vi "Quadro.vi"() -> ()   [LabVIEW 2012]
panel:
  out "Kąt x 2":u32
  out "Kąt x":u32
  out "Kąt y 2":u32
  out "Kąt y":u32
  out "Kąt z 2":u32
  out "Kąt z":u32
  out "x+y":u16
  out "Array":u8[](array[numeric])
  in  "Stop":bool
  out "error out":errorcluster
  in  "Opóźnienie pętli [ms]":u32
  in  "Czas oczekiwania po wysłaniu [ms]":u32
  in  "Dane wysłane":string="d"
  out "Nazwa urządzenia":string
  in  "Limit czasu - bluetooth [ms]":i32=1000
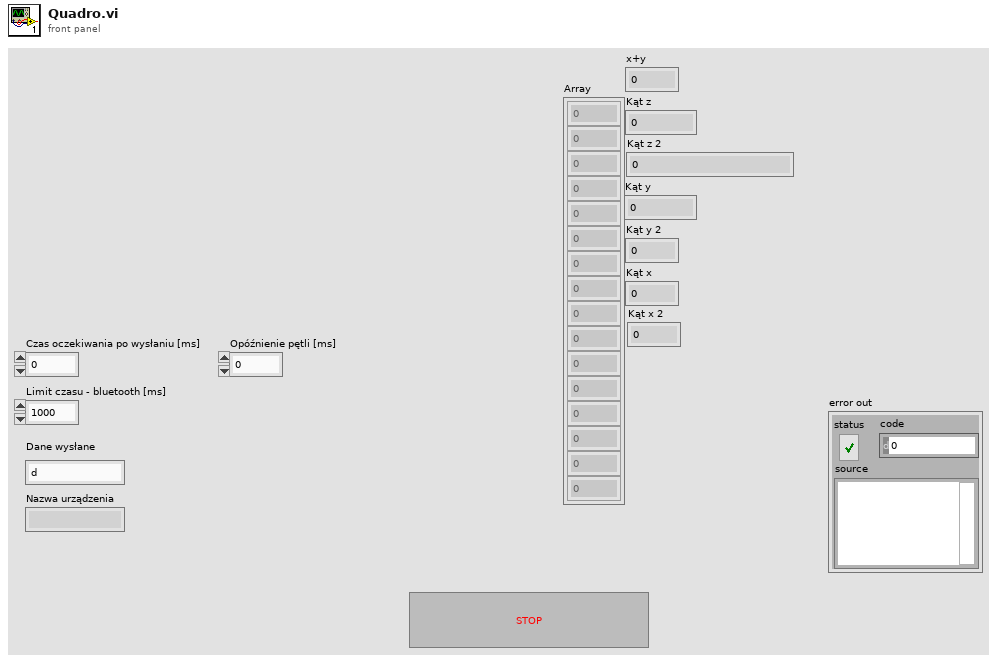
[diagram p1: front panel]
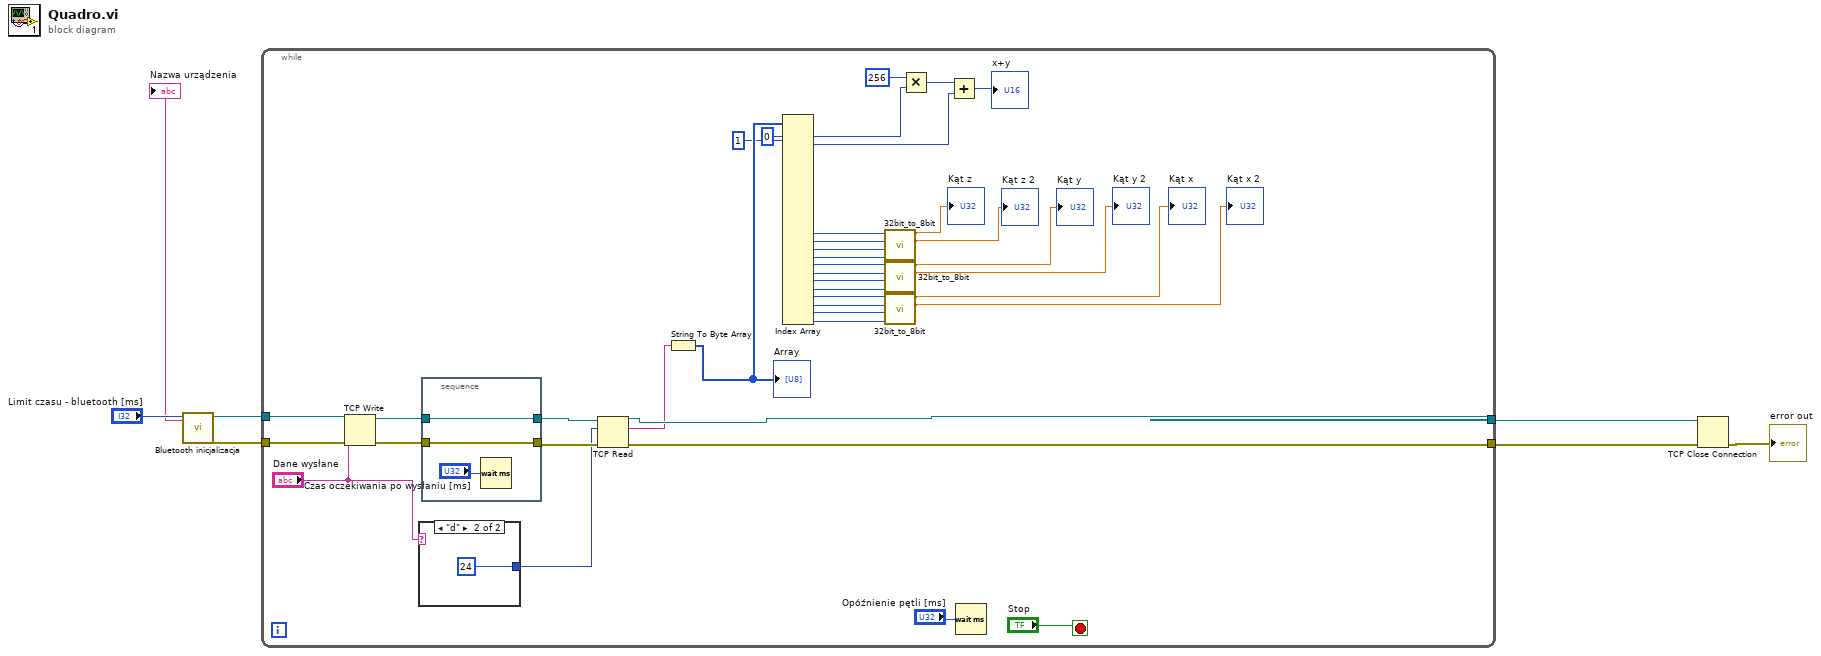
[diagram p0: block diagram]
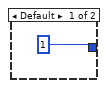
[diagram p2: hidden frame]
diagram:
  n1 = call "Bluetooth inicjalizacja.vi"("time limit ms (10000)"="Limit czasu - bluetooth [ms]") -> ("error out"=w4:errorcluster, "Bluetooth Network Connection out"=w5:refnum<k31>, "Device Name"=→"Nazwa urządzenia":string)  [unwired: 5 in, 3 out]
  n2 = while {
    tunnel: w5 -> [w46]
    tunnel: w4 -> [w45]
    tunnel: [w39] -> w2
    tunnel: [w37] -> w1
    stop <- "Stop" stop-if-true
    n3 = TCP Write(connection ID=w46, data in="Dane wysłane", error in (no error)=w45) -> (connection ID out=w44:refnum<k31>, error out=w43:errorcluster)  [unwired: 1 in, 1 out]
    n4 = case shown="\"d\"" "Dane wysłane" {
      tunnel: [1 24 ("bytes to read")] -> w34
      frame Default {
      }
      frame "d" {
      }
    }
    n5 = stacked-sequence "Waiting time" {
      tunnel: [w50] -> w42
      tunnel: w44 -> [w50]
      tunnel: [w49] -> w41
      tunnel: w43 -> [w49]
      frame #0 {
        n6 = Wait (ms)(milliseconds to wait="Czas oczekiwania po wysłaniu [ms]") -> ()  [unwired: 1 out]
      }
    }
    n7 = TCP Read(connection ID=w42, bytes to read=w34, error in (no error)=w41) -> (connection ID out=w39:refnum<k31>, data out=w36:string, error out=w37:errorcluster)  [unwired: 2 in]
    n8 = String To Byte Array(string=w36) -> (unsigned byte array=w33:u8[])
    "Array" <- w33
    n9 = Index Array(array=w33, index #1=0 ("index"), index #2=1 ("index")) -> (element #1=w31:u8, element #2=w28:u8, element #13=w25:u8, element #14=w24:u8, element #15=w23:u8, element #16=w22:u8, element #17=w21:u8, element #18=w20:u8, element #19=w19:u8, element #20=w18:u8, element #21=w17:u8, element #22=w16:u8, element #23=w15:u8, element #24=w14:u8)  [unwired: 22 in, 10 out]
    n10 = call "32bit_to_8bit.vi"("Numeric 6"=w22, "Numeric 5"=w23, "Numeric 4"=w24, "Numeric in"=w25) -> ("Numeric out"=→"Kąt z 2":dbl, "Numeric 3"=→"Kąt z":dbl)  [unwired: 6 in]
    n11 = call "32bit_to_8bit.vi"("Numeric 6"=w18, "Numeric 5"=w19, "Numeric 4"=w20, "Numeric in"=w21) -> ("Numeric out"=→"Kąt y 2":dbl, "Numeric 3"=→"Kąt y":dbl)  [unwired: 6 in]
    n12 = call "32bit_to_8bit.vi"("Numeric 6"=w14, "Numeric 5"=w15, "Numeric 4"=w16, "Numeric in"=w17) -> ("Numeric out"=→"Kąt x 2":dbl, "Numeric 3"=→"Kąt x":dbl)  [unwired: 6 in]
    n13 = Multiply(x=u16 256, y=w31) -> (x*y=w29:u16)
    n14 = Add(x=w29, y=w28) -> (x+y=→"x+y":u16)
    n15 = Wait (ms)(milliseconds to wait="Opóźnienie pętli [ms]") -> ()  [unwired: 1 out]
  }
  n16 = TCP Close Connection(connection ID=w2, error in (no error)=w1) -> (error out=→"error out":errorcluster)  [unwired: 1 in, 1 out]
